vi "check caen global enable.vi"(8 "error in":errorcluster, 11 "VISA in":refnum<visa-resource-name>) -> (0 "error out":errorcluster, 2 "CAEN Global HV Enable":bool, 3 "VISA out":refnum<visa-resource-name>)   [LabVIEW 2018]
uses:
  archive/CAEN_SY527 v3/CAEN_SY527/subvis/set location.ctl
  archive/CAEN_SY527 v3/CAEN_SY527/CAEN globals.vi
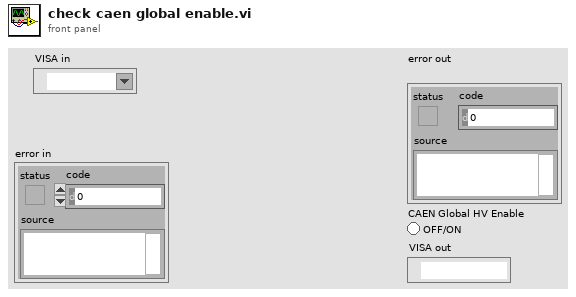
[diagram p1: front panel]
types:
  T1 = typedef "set location.ctl" = cluster{"set index":i32, "set Screen":string, "set subpage":i32, "set column":i32, "Group":string, "Crate":i32}
  T2 = typedef "location cluster.ctl" = cluster{"Column":i32, "Card Type":string, "Channel":i32, "Card":i32, "Default response":string, "Entering":string, "Entering state":bool, "subpage":i32, "page":i32, "Crate":i32, "Screen":string, "Group":string, "Global HV Enable":bool}
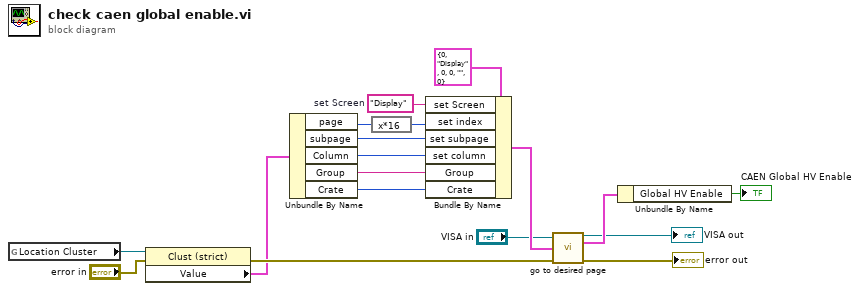
[diagram p0: block diagram]
diagram:
  w7 = "Display"  # set Screen
  n1 = global read "CAEN globals.vi" "Location Cluster"() -> (w18:refnum<vi>)
  n2 = property class="Clust (strict)"(reference=w18, error in="error in") -> (error out=w16:errorcluster, "Value"=w15:T2)  [unwired: 1 out]
  n3 = Unbundle By Name(w15) -> ("page"=w8:i32, "subpage"=w10:i32, "Column"=w11:i32, "Group"=w12:string, "Crate"=w13:i32)
  n4 = expression code="x*16"(w8) -> (w9:i32)
  n5 = Bundle By Name(cluster=T1 {"set index"=0, "set Screen"="Display", "set subpage"=0, "set column"=0, "Group"="", "Crate"=0} ("Set Cluster"), "set Screen"=w7, "set index"=w9, "set subpage"=w10, "set column"=w11, "Group"=w12, "Crate"=w13) -> (w6:T1)
  n6 = call "go to desired page.vi"("VISA in"="VISA in", "Set Cluster"=w6, "error in"=w16) -> ("VISA out"=→"VISA out":refnum<visa-resource-name>, "Location Cluster out"=w5:T2, "error out"=→"error out":errorcluster)  [unwired: 9 in, 1 out]
  n7 = Unbundle By Name(w5) -> ("Global HV Enable"=→"CAEN Global HV Enable":bool)
